vi "Extend.vi"(6 "Step":dbl, 8 "enemy_robots":T1[](array[typedef]), 10 "Target":dbl[](array[numeric]), 11 "Nearest":dbl[](array[numeric])) -> (2 "New State":dbl[](array[numeric]))   [LabVIEW 2017]
uses:
  Core/AI Robot.ctl
  Intel/Functions Enum.ctl
  Intel/AttackerStates.ctl
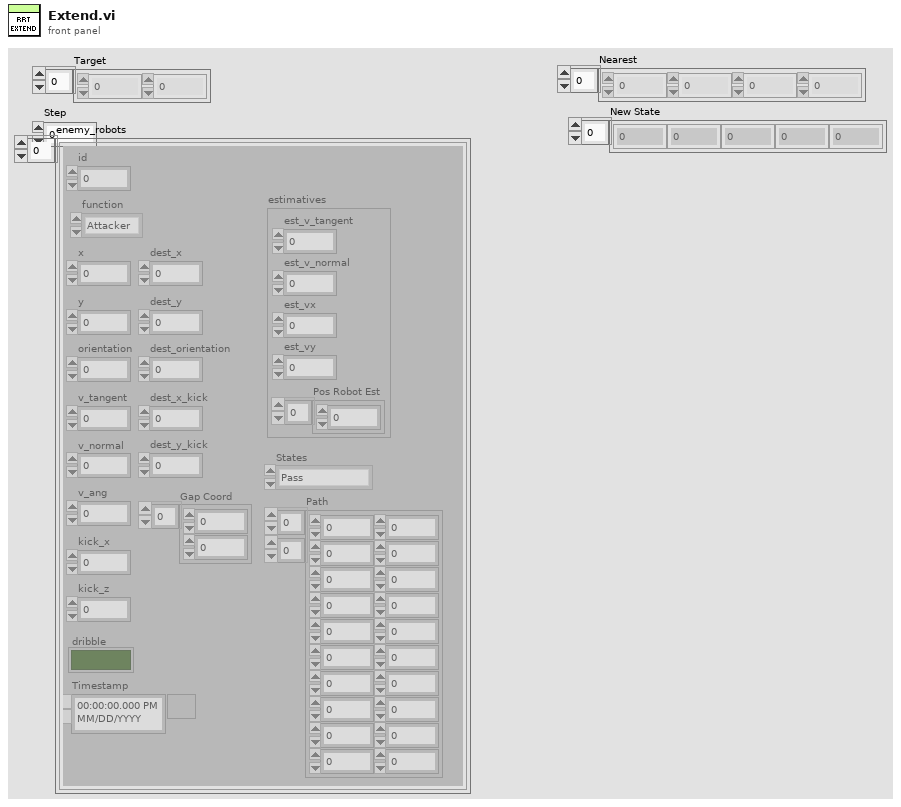
[diagram p1: front panel]
types:
  T1 = typedef "AI Robot.ctl" = cluster{"id":u32, "function":T2, "x":dbl, "y":dbl, "orientation":dbl, "v_tangent":dbl, "v_normal":dbl, "v_ang":dbl, "kick_x":dbl, "kick_z":dbl, "dribble":bool, "Timestamp":timestamp, "dest_x":dbl, "dest_y":dbl, "dest_orientation":dbl, "estimatives":cluster{"est_v_tangent":dbl, "est_v_normal":dbl, "est_vx":dbl, "est_vy":dbl, "Pos Robot Est":dbl[]}, "dest_x_kick":dbl, "dest_y_kick":dbl, "Gap Coord":dbl[], "States":T3, "Path ":dbl[][]}
  T2 = typedef "Functions Enum.ctl" = enum16{"Attacker", "Goalie", "Defender", "Striker", "Goto 0", "Dummy", "Kicker", "ZigZag"}
  T3 = typedef "AttackerStates.ctl" = enum16{"Pass", "GoToTangent", "BallGetting", "GoToKick", ""}
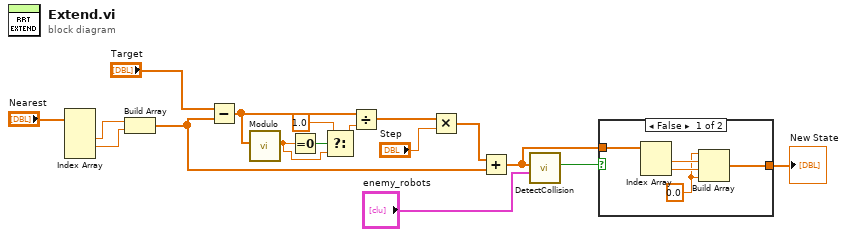
[diagram p0: block diagram]
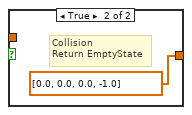
[diagram p2: hidden frame]
diagram:
  n1 = Index Array(array="Nearest") -> (element #2=w7:dbl, element #3=w6:dbl)  [unwired: 4 in, 2 out]
  n2 = Build Array(w7, w6) -> (w5:dbl[])
  n3 = Subtract(x="Target", y=w5) -> (x-y=w16:dbl[])
  n4 = call "Modulo.vi"("2D vector"=w16) -> ("Modulo"=w1:dbl)  [unwired: 10 in]
  n5 = Equal To 0?(x=w1) -> (x = 0?=w3:bool)
  n6 = Select(t=1.0, s=w3, f=w1) -> (s? t:f=w4:dbl)
  n7 = Divide(x=w16, y=w4) -> (x/y=w15:dbl[])
  n8 = Multiply(x=w15, y="Step") -> (x*y=w13:dbl[])
  n9 = Add(x=w13, y=w5) -> (x+y=w10:dbl[])
  n10 = call "DetectCollision.vi"("enemy_robots"="enemy_robots", "Point"=w10) -> ("Collision"=w11:bool)  [unwired: 9 in]
  n11 = case shown="False" w11 {
    tunnel: [w18 dbl[] [0.0, 0.0, 0.0, -1.0] ("Nearest")] -> w9
    tunnel: w10 -> [w22 _]
    frame False {
      w19 = 0.0 ("element")
      n12 = Index Array(array=w22) -> (element #1=w21:dbl, element #2=w20:dbl)  [unwired: 2 in]
      n13 = Build Array(w19, w21, w20, w19) -> (w18:dbl[])
    }
    frame True {
      # "Collision\nReturn EmptyState"
    }
  }
  "New State" <- w9
